vi "Close Occupancy Grid Map.vi"(8 "error in (no error)":errorcluster, 11 "map reference in":refnum<data-value>) -> (0 "error out":errorcluster)   [LabVIEW 2017, in "NI_Robotics_OccupancyGridWorldMap.lvclass"]
doc: "Closes an open reference to an occupancy grid map object."
uses:
  <vilib>/robotics/Navigation/shared/WorldMap/OccupancyGridWorldMap/NI_Robotics_OccupancyGridWorldMap.lvclass
  <vilib>/robotics/Navigation/shared/WorldMap/OccupancyGridWorldMap/NI_Robotics_OccupancyGridWorldMap.lvclass/NI_Robotics_OccupancyGridWorldMap.ctl
  <vilib>/robotics/Navigation/shared/MapNode/OccupancyGridNode/NI_Robotics_OccupancyGridMapNode.lvclass
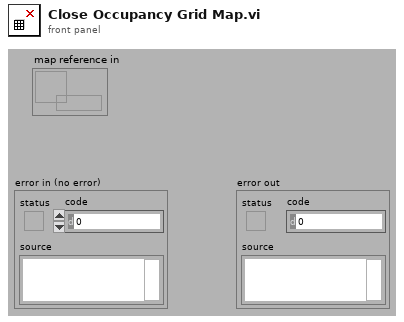
[diagram p1: front panel]
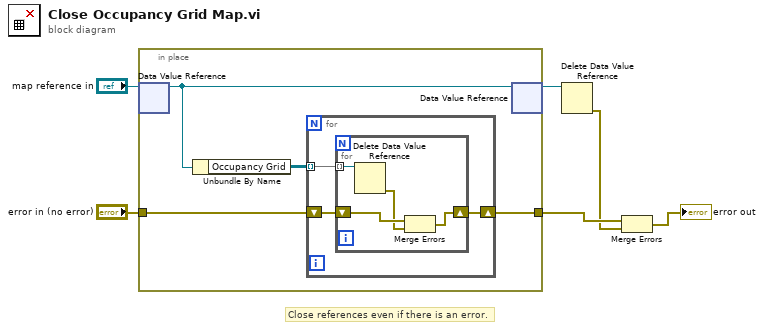
[diagram p0: block diagram]
diagram:
  # "Close references even if there is an error."
  n1 = in-place {
    in-place-border: "error in (no error)" -> [w7]
    in-place-border: [w10] -> w3
    n2 = in-place-dvr #1("map reference in") -> (w9:refnum<class "NI_Robotics_OccupancyGridWorldMap.lvclass">)  [unwired: 1 out]
    n3 = Unbundle By Name(w9) -> ("Occupancy Grid"=w8:refnum<data-value>[][])
    n4 = for {
      shift-right: [w13] -> w10
      shift-left: w7 -> [w12]
      tunnel: w8 -> [w11] mode=indexing
      n5 = for {
        shift-right: [w14] -> w13
        shift-left: w12 -> [w16]
        tunnel: w11 -> [w17] mode=indexing
        n6 = Delete Data Value Reference(data value reference=w17) -> (error out=w15:errorcluster)  [unwired: 1 in, 1 out]
        n7 = Merge Errors(w16, w15) -> (w14:errorcluster)
      }
    }
    n8 = in-place-dvr #1(w9) -> (w4:refnum<data-value>)  [unwired: 1 out]
  }
  n9 = Delete Data Value Reference(data value reference=w4) -> (error out=w2:errorcluster)  [unwired: 1 in, 1 out]
  n10 = Merge Errors(w3, w2) -> (→"error out":errorcluster)
